vi "Anritsu_MT8852B_YYLL_SetResultVar.vi"(8 "error in (no error)":errorcluster, 9 "Anritsu_MT8852B_YYLL_Result":T1={"AnritsuMT8852B_OP_Low_Avgpower"=-9999.0, "AnritsuMT8852B_OP_Low_Peakpower"=-9999.0, "AnritsuMT8852B_OP_Med_Avgpower"=-9999.0, "AnritsuMT8852B_OP_Med_Peakpower"=-9999.0, "AnritsuMT8852B_OP_Hig_Avgpower"=-9999.0, "AnritsuMT8852B_OP_Hig_Peakpower"=-9999.0, "AnritsuMT8852B_IC_Low_PositiveOffset"=-9999.0, "AnritsuMT8852B_IC_Low_NegativeOffset"=-9999.0, "AnritsuMT8852B_IC_Low_AvgOffset"=-9999.0, "AnritsuMT8852B_IC_Med_PositiveOffset"=-9999.0, "AnritsuMT8852B_IC_Med_NegativeOffset"=-9999.0, "AnritsuMT8852B_IC_Med_AvgOffset"=-9999.0, "AnritsuMT8852B_IC_Hig_PositiveOffset"=-9999.0, "AnritsuMT8852B_IC_Hig_NegativeOffset"=-9999.0, "AnritsuMT8852B_IC_Hig_AvgOffset"=-9999.0, "AnritsuMT8852B_SS_Low_BitErrorRate"=-9999.0, "AnritsuMT8852B_SS_Low_FrameErrorRate"=-9999.0, "AnritsuMT8852B_SS_Med_BitErrorRate"=-9999.0, "AnritsuMT8852B_SS_Med_FrameErrorRate"=-9999.0, "AnritsuMT8852B_SS_Hig_BitErrorRate"=-9999.0, "AnritsuMT8852B_SS_Hig_FrameErrorRate"=-9999.0, "StandardLim_OP_Avg[-6,20]"=FALSE, "StandardLim_OP_Peak[<23]"=FALSE, "StandardLim_IC_Offset[75KHz]"=FALSE, "StandardLim_SS_BitErrorRate[<0.1]"=FALSE, "StandardLim_SS_FrameErrorRate[<100]"=FALSE}, 11 "函数池名称":i32) -> (0 "error out":errorcluster)   [LabVIEW 2017]
uses:
  Anritsu_MT8852B_YYLL_Result.ctl
  YYLLGeneric/variable_W.ctl
  YtCommon.lvlibp/yt`Data-Ytester Type Data.ctl
  YtCommon.lvlibp
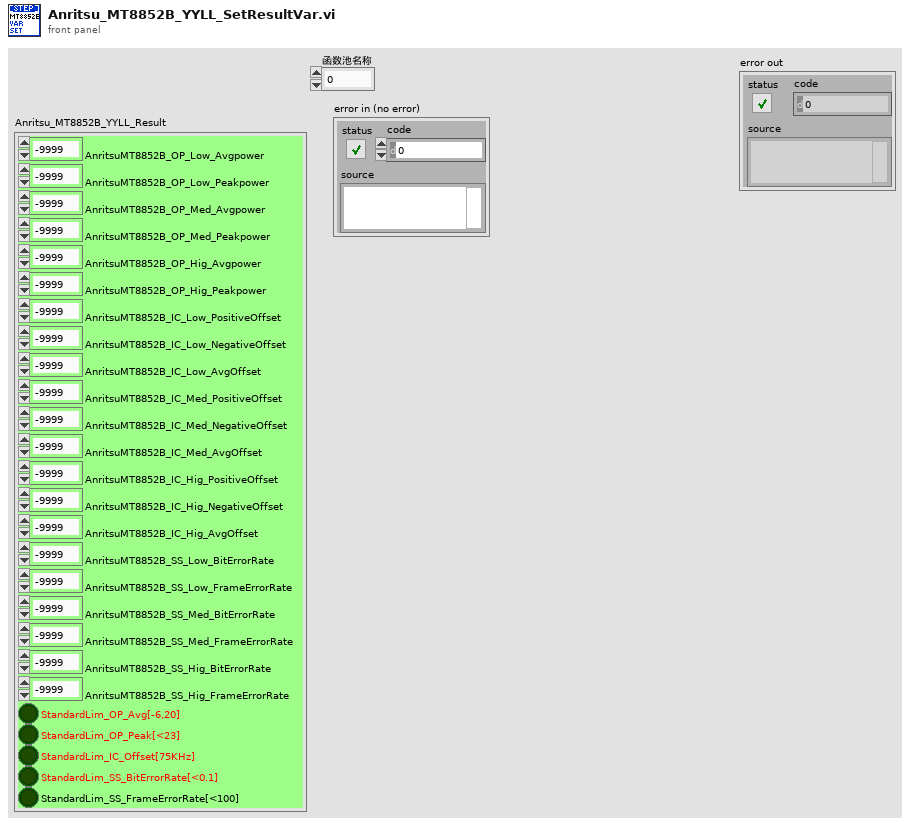
[diagram p1: front panel]
types:
  T1 = typedef "Anritsu_MT8852B_YYLL_Result.ctl" = cluster{"AnritsuMT8852B_OP_Low_Avgpower":dbl, "AnritsuMT8852B_OP_Low_Peakpower":dbl, "AnritsuMT8852B_OP_Med_Avgpower":dbl, "AnritsuMT8852B_OP_Med_Peakpower":dbl, "AnritsuMT8852B_OP_Hig_Avgpower":dbl, "AnritsuMT8852B_OP_Hig_Peakpower":dbl, "AnritsuMT8852B_IC_Low_PositiveOffset":dbl, "AnritsuMT8852B_IC_Low_NegativeOffset":dbl, "AnritsuMT8852B_IC_Low_AvgOffset":dbl, "AnritsuMT8852B_IC_Med_PositiveOffset":dbl, "AnritsuMT8852B_IC_Med_NegativeOffset":dbl, "AnritsuMT8852B_IC_Med_AvgOffset":dbl, "AnritsuMT8852B_IC_Hig_PositiveOffset":dbl, "AnritsuMT8852B_IC_Hig_NegativeOffset":dbl, "AnritsuMT8852B_IC_Hig_AvgOffset":dbl, "AnritsuMT8852B_SS_Low_BitErrorRate":dbl, "AnritsuMT8852B_SS_Low_FrameErrorRate":dbl, "AnritsuMT8852B_SS_Med_BitErrorRate":dbl, "AnritsuMT8852B_SS_Med_FrameErrorRate":dbl, "AnritsuMT8852B_SS_Hig_BitErrorRate":dbl, "AnritsuMT8852B_SS_Hig_FrameErrorRate":dbl, "StandardLim_OP_Avg[-6,20]":bool, "StandardLim_OP_Peak[<23]":bool, "StandardLim_IC_Offset[75KHz]":bool, "StandardLim_SS_BitErrorRate[<0.1]":bool, "StandardLim_SS_FrameErrorRate[<100]":bool}
  T2 = typedef "variable_W.ctl" = cluster{"YT_TYPE":T3, "TypeData":string[], "Tips":string}
  T3 = typedef "YtCommon.lvlibp/yt`Data-Ytester Type Data.ctl" = enum16{"NULL", "NUM", "BOOL", "TXT", "ENUM", "TIME", "PATH", "VISA", "COMBO", "ColorBox", "RadioBtn", "Array_NUM", "Array_BOOL", "Array_TXT", "Array_ENUM", "Array_PATH", "Array_COMBO"}
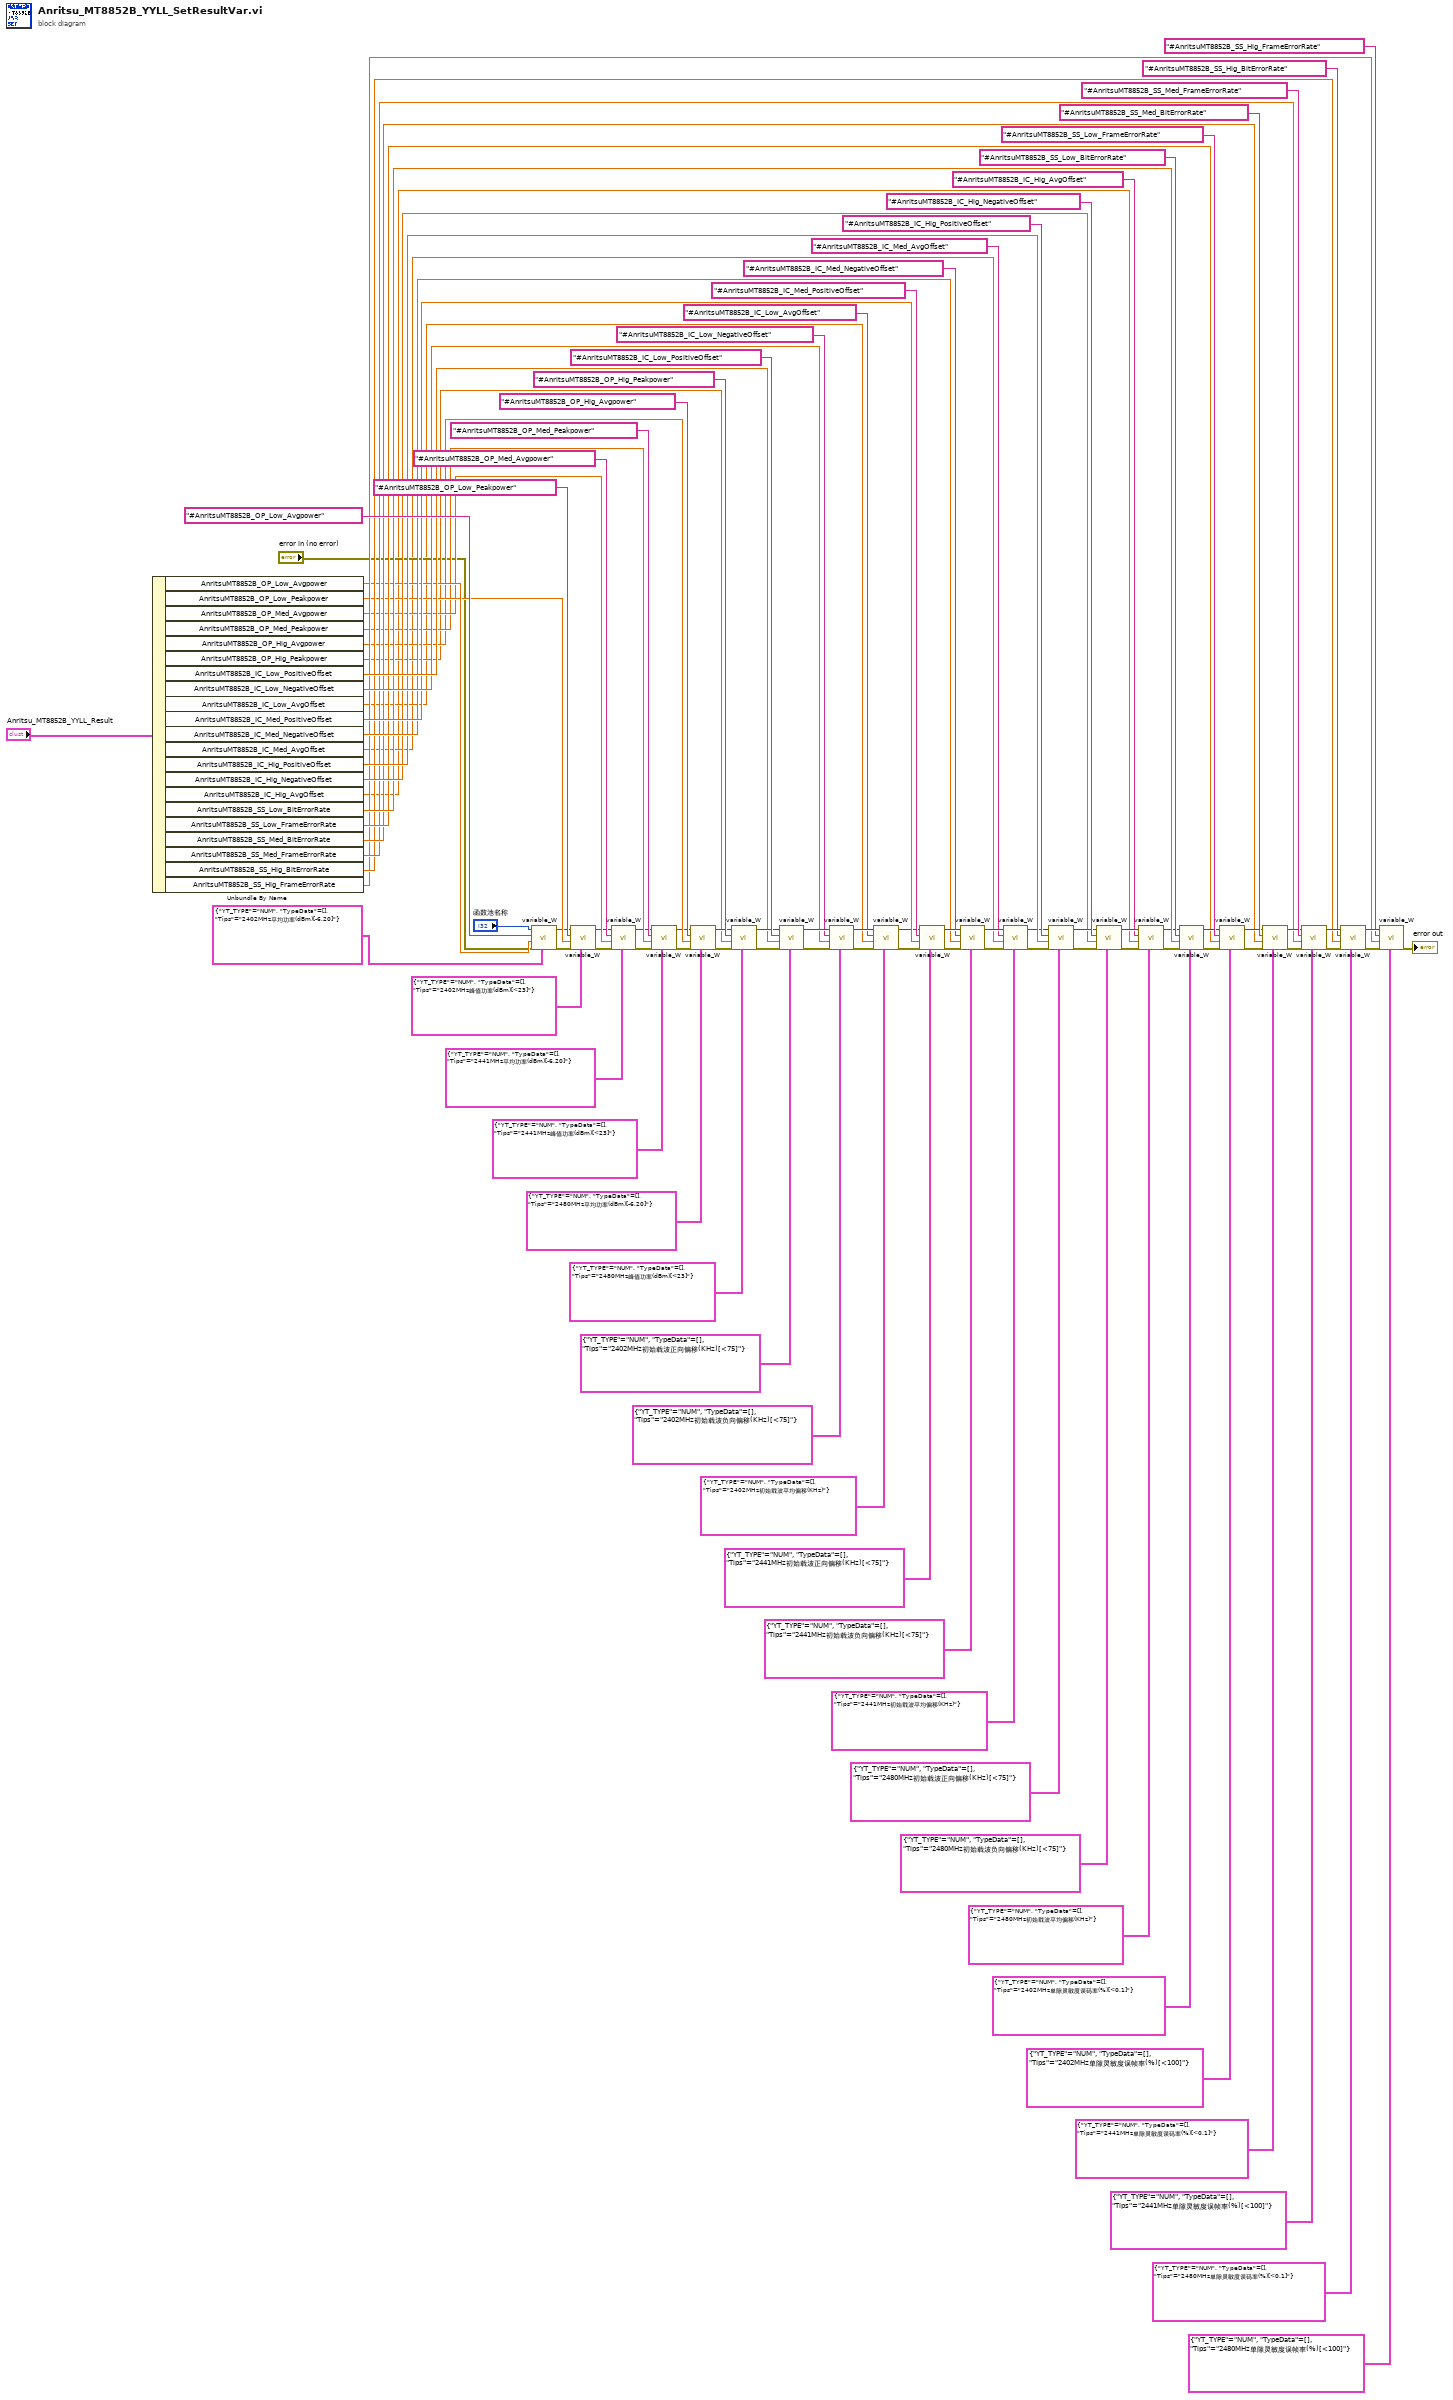
[diagram p0: block diagram]
diagram:
  n1 = Unbundle By Name("Anritsu_MT8852B_YYLL_Result") -> ("AnritsuMT8852B_OP_Low_Avgpower"=w39:dbl, "AnritsuMT8852B_OP_Low_Peakpower"=w38:dbl, "AnritsuMT8852B_OP_Med_Avgpower"=w36:dbl, "AnritsuMT8852B_OP_Med_Peakpower"=w34:dbl, "AnritsuMT8852B_OP_Hig_Avgpower"=w32:dbl, "AnritsuMT8852B_OP_Hig_Peakpower"=w29:dbl, "AnritsuMT8852B_IC_Low_PositiveOffset"=w51:dbl, "AnritsuMT8852B_IC_Low_NegativeOffset"=w50:dbl, "AnritsuMT8852B_IC_Low_AvgOffset"=w6:dbl, "AnritsuMT8852B_IC_Med_PositiveOffset"=w49:dbl, "AnritsuMT8852B_IC_Med_NegativeOffset"=w48:dbl, "AnritsuMT8852B_IC_Med_AvgOffset"=w5:dbl, "AnritsuMT8852B_IC_Hig_PositiveOffset"=w47:dbl, "AnritsuMT8852B_IC_Hig_NegativeOffset"=w46:dbl, "AnritsuMT8852B_IC_Hig_AvgOffset"=w4:dbl, "AnritsuMT8852B_SS_Low_BitErrorRate"=w45:dbl, "AnritsuMT8852B_SS_Low_FrameErrorRate"=w44:dbl, "AnritsuMT8852B_SS_Med_BitErrorRate"=w43:dbl, "AnritsuMT8852B_SS_Med_FrameErrorRate"=w42:dbl, "AnritsuMT8852B_SS_Hig_BitErrorRate"=w41:dbl, "AnritsuMT8852B_SS_Hig_FrameErrorRate"=w40:dbl)
  n2 = call "variable_W.vi"("附加的Information"=T2 {"YT_TYPE"=enum."NUM", "TypeData"=[], "Tips"="2402MHz平均功率(dBm)[-6,20]"}, "error in (no error)"="error in (no error)", "待写入池的输入控件"=w39, "待写入池变量名称"="#AnritsuMT8852B_OP_Low_Avgpower", "函数池名称 in"="函数池名称") -> ("error out"=w24:errorcluster, "函数池名称 out"=w37:i32)  [unwired: 4 in, 1 out]
  n3 = call "variable_W.vi"("附加的Information"=T2 {"YT_TYPE"=enum."NUM", "TypeData"=[], "Tips"="2402MHz峰值功率(dBm)[<23]"}, "error in (no error)"=w24, "待写入池的输入控件"=w38, "待写入池变量名称"="#AnritsuMT8852B_OP_Low_Peakpower", "函数池名称 in"=w37) -> ("error out"=w25:errorcluster, "函数池名称 out"=w35:i32)  [unwired: 4 in, 1 out]
  n4 = call "variable_W.vi"("附加的Information"=T2 {"YT_TYPE"=enum."NUM", "TypeData"=[], "Tips"="2441MHz平均功率(dBm)[-6,20]"}, "error in (no error)"=w25, "待写入池的输入控件"=w36, "待写入池变量名称"="#AnritsuMT8852B_OP_Med_Avgpower", "函数池名称 in"=w35) -> ("error out"=w26:errorcluster, "函数池名称 out"=w33:i32)  [unwired: 4 in, 1 out]
  n5 = call "variable_W.vi"("附加的Information"=T2 {"YT_TYPE"=enum."NUM", "TypeData"=[], "Tips"="2441MHz峰值功率(dBm)[<23]"}, "error in (no error)"=w26, "待写入池的输入控件"=w34, "待写入池变量名称"="#AnritsuMT8852B_OP_Med_Peakpower", "函数池名称 in"=w33) -> ("error out"=w27:errorcluster, "函数池名称 out"=w31:i32)  [unwired: 4 in, 1 out]
  n6 = call "variable_W.vi"("附加的Information"=T2 {"YT_TYPE"=enum."NUM", "TypeData"=[], "Tips"="2480MHz平均功率(dBm)[-6,20]"}, "error in (no error)"=w27, "待写入池的输入控件"=w32, "待写入池变量名称"="#AnritsuMT8852B_OP_Hig_Avgpower", "函数池名称 in"=w31) -> ("error out"=w28:errorcluster, "函数池名称 out"=w30:i32)  [unwired: 4 in, 1 out]
  n7 = call "variable_W.vi"("附加的Information"=T2 {"YT_TYPE"=enum."NUM", "TypeData"=[], "Tips"="2480MHz峰值功率(dBm)[<23]"}, "error in (no error)"=w28, "待写入池的输入控件"=w29, "待写入池变量名称"="#AnritsuMT8852B_OP_Hig_Peakpower", "函数池名称 in"=w30) -> ("error out"=w60:errorcluster, "函数池名称 out"=w61:i32)  [unwired: 4 in, 1 out]
  n8 = call "variable_W.vi"("附加的Information"=T2 {"YT_TYPE"=enum."NUM", "TypeData"=[], "Tips"="2402MHz初始载波正向偏移(KHz)[<75]"}, "error in (no error)"=w60, "待写入池的输入控件"=w51, "待写入池变量名称"="#AnritsuMT8852B_IC_Low_PositiveOffset", "函数池名称 in"=w61) -> ("error out"=w59:errorcluster, "函数池名称 out"=w85:i32)  [unwired: 4 in, 1 out]
  n9 = call "variable_W.vi"("附加的Information"=T2 {"YT_TYPE"=enum."NUM", "TypeData"=[], "Tips"="2402MHz初始载波负向偏移(KHz)[<75]"}, "error in (no error)"=w59, "待写入池的输入控件"=w50, "待写入池变量名称"="#AnritsuMT8852B_IC_Low_NegativeOffset", "函数池名称 in"=w85) -> ("error out"=w23:errorcluster, "函数池名称 out"=w22:i32)  [unwired: 4 in, 1 out]
  n10 = call "variable_W.vi"("附加的Information"=T2 {"YT_TYPE"=enum."NUM", "TypeData"=[], "Tips"="2402MHz初始载波平均偏移(KHz)"}, "error in (no error)"=w23, "待写入池的输入控件"=w6, "待写入池变量名称"="#AnritsuMT8852B_IC_Low_AvgOffset", "函数池名称 in"=w22) -> ("error out"=w21:errorcluster, "函数池名称 out"=w20:i32)  [unwired: 4 in, 1 out]
  n11 = call "variable_W.vi"("附加的Information"=T2 {"YT_TYPE"=enum."NUM", "TypeData"=[], "Tips"="2441MHz初始载波正向偏移(KHz)[<75]"}, "error in (no error)"=w21, "待写入池的输入控件"=w49, "待写入池变量名称"="#AnritsuMT8852B_IC_Med_PositiveOffset", "函数池名称 in"=w20) -> ("error out"=w58:errorcluster, "函数池名称 out"=w93:i32)  [unwired: 4 in, 1 out]
  n12 = call "variable_W.vi"("附加的Information"=T2 {"YT_TYPE"=enum."NUM", "TypeData"=[], "Tips"="2441MHz初始载波负向偏移(KHz)[<75]"}, "error in (no error)"=w58, "待写入池的输入控件"=w48, "待写入池变量名称"="#AnritsuMT8852B_IC_Med_NegativeOffset", "函数池名称 in"=w93) -> ("error out"=w13:errorcluster, "函数池名称 out"=w19:i32)  [unwired: 4 in, 1 out]
  n13 = call "variable_W.vi"("附加的Information"=T2 {"YT_TYPE"=enum."NUM", "TypeData"=[], "Tips"="2441MHz初始载波平均偏移(KHz)"}, "error in (no error)"=w13, "待写入池的输入控件"=w5, "待写入池变量名称"="#AnritsuMT8852B_IC_Med_AvgOffset", "函数池名称 in"=w19) -> ("error out"=w12:errorcluster, "函数池名称 out"=w18:i32)  [unwired: 4 in, 1 out]
  n14 = call "variable_W.vi"("附加的Information"=T2 {"YT_TYPE"=enum."NUM", "TypeData"=[], "Tips"="2480MHz初始载波正向偏移(KHz)[<75]"}, "error in (no error)"=w12, "待写入池的输入控件"=w47, "待写入池变量名称"="#AnritsuMT8852B_IC_Hig_PositiveOffset", "函数池名称 in"=w18) -> ("error out"=w57:errorcluster, "函数池名称 out"=w86:i32)  [unwired: 4 in, 1 out]
  n15 = call "variable_W.vi"("附加的Information"=T2 {"YT_TYPE"=enum."NUM", "TypeData"=[], "Tips"="2480MHz初始载波负向偏移(KHz)[<75]"}, "error in (no error)"=w57, "待写入池的输入控件"=w46, "待写入池变量名称"="#AnritsuMT8852B_IC_Hig_NegativeOffset", "函数池名称 in"=w86) -> ("error out"=w15:errorcluster, "函数池名称 out"=w17:i32)  [unwired: 4 in, 1 out]
  n16 = call "variable_W.vi"("附加的Information"=T2 {"YT_TYPE"=enum."NUM", "TypeData"=[], "Tips"="2480MHz初始载波平均偏移(KHz)"}, "error in (no error)"=w15, "待写入池的输入控件"=w4, "待写入池变量名称"="#AnritsuMT8852B_IC_Hig_AvgOffset", "函数池名称 in"=w17) -> ("error out"=w14:errorcluster, "函数池名称 out"=w16:i32)  [unwired: 4 in, 1 out]
  n17 = call "variable_W.vi"("附加的Information"=T2 {"YT_TYPE"=enum."NUM", "TypeData"=[], "Tips"="2402MHz单隙灵敏度误码率(%)[<0.1]"}, "error in (no error)"=w14, "待写入池的输入控件"=w45, "待写入池变量名称"="#AnritsuMT8852B_SS_Low_BitErrorRate", "函数池名称 in"=w16) -> ("error out"=w56:errorcluster, "函数池名称 out"=w72:i32)  [unwired: 4 in, 1 out]
  n18 = call "variable_W.vi"("附加的Information"=T2 {"YT_TYPE"=enum."NUM", "TypeData"=[], "Tips"="2402MHz单隙灵敏度误帧率(%)[<100]"}, "error in (no error)"=w56, "待写入池的输入控件"=w44, "待写入池变量名称"="#AnritsuMT8852B_SS_Low_FrameErrorRate", "函数池名称 in"=w72) -> ("error out"=w55:errorcluster, "函数池名称 out"=w71:i32)  [unwired: 4 in, 1 out]
  n19 = call "variable_W.vi"("附加的Information"=T2 {"YT_TYPE"=enum."NUM", "TypeData"=[], "Tips"="2441MHz单隙灵敏度误码率(%)[<0.1]"}, "error in (no error)"=w55, "待写入池的输入控件"=w43, "待写入池变量名称"="#AnritsuMT8852B_SS_Med_BitErrorRate", "函数池名称 in"=w71) -> ("error out"=w54:errorcluster, "函数池名称 out"=w62:i32)  [unwired: 4 in, 1 out]
  n20 = call "variable_W.vi"("附加的Information"=T2 {"YT_TYPE"=enum."NUM", "TypeData"=[], "Tips"="2441MHz单隙灵敏度误帧率(%)[<100]"}, "error in (no error)"=w54, "待写入池的输入控件"=w42, "待写入池变量名称"="#AnritsuMT8852B_SS_Med_FrameErrorRate", "函数池名称 in"=w62) -> ("error out"=w53:errorcluster, "函数池名称 out"=w69:i32)  [unwired: 4 in, 1 out]
  n21 = call "variable_W.vi"("附加的Information"=T2 {"YT_TYPE"=enum."NUM", "TypeData"=[], "Tips"="2480MHz单隙灵敏度误码率(%)[<0.1]"}, "error in (no error)"=w53, "待写入池的输入控件"=w41, "待写入池变量名称"="#AnritsuMT8852B_SS_Hig_BitErrorRate", "函数池名称 in"=w69) -> ("error out"=w52:errorcluster, "函数池名称 out"=w70:i32)  [unwired: 4 in, 1 out]
  n22 = call "variable_W.vi"("附加的Information"=T2 {"YT_TYPE"=enum."NUM", "TypeData"=[], "Tips"="2480MHz单隙灵敏度误帧率(%)[<100]"}, "error in (no error)"=w52, "待写入池的输入控件"=w40, "待写入池变量名称"="#AnritsuMT8852B_SS_Hig_FrameErrorRate", "函数池名称 in"=w70) -> ("error out"=→"error out":errorcluster)  [unwired: 4 in, 2 out]
